vi "Parse Profile Status Response.vi"(8 "error in (no error)":errorcluster, 11 "Profile Status":string[](array[string])) -> (0 "error out":errorcluster, 3 "Profile Status":T1={"Profile State"=enum."Not Running", "Current Profile"=0, "Total Time Remaining"=0, "Total Steps"=0})   [LabVIEW 2018, in "F4T.lvlib" / "F4T.lvclass"]
uses:
  F4T.lvclass
  PPLs/Temp Chamber/Parent/Temp Chamber.lvlibp/Custom Controls/Profile Status.ctl
  PPLs/Temp Chamber/Parent/Temp Chamber.lvlibp/Custom Controls/Profile State.ctl
  PPLs/Temp Chamber/Parent/Temp Chamber.lvlibp/Temp Chamber.lvclass
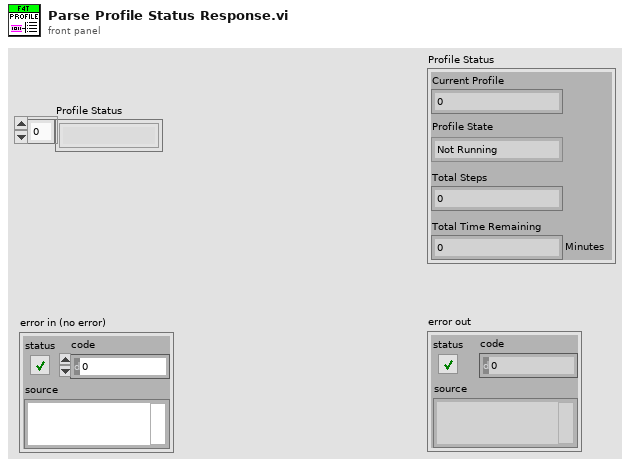
[diagram p1: front panel]
types:
  T1 = typedef "Temp Chamber.lvlibp/Temp Chamber.lvclass/Profile Status.ctl" = cluster{"Profile State":T2, "Current Profile":u32, "Total Time Remaining":u32, "Total Steps":u32}
  T2 = typedef "Temp Chamber.lvlibp/Temp Chamber.lvclass/Profile State.ctl" = enum16{"Running", "Not Running", "Paused", "Completed", "Terminated"}
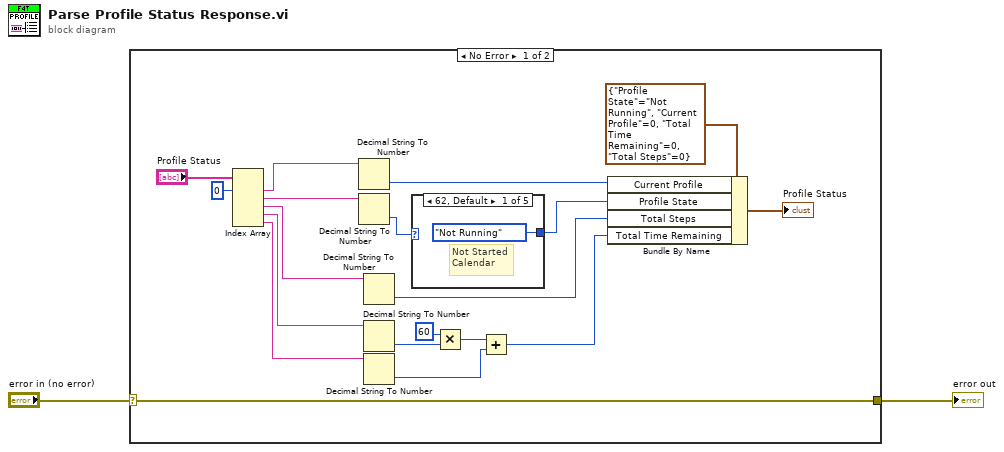
[diagram p0: block diagram]
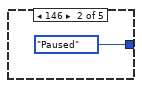
[diagram p2: hidden frame]
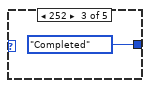
[diagram p3: hidden frame]
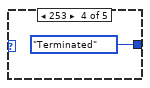
[diagram p4: hidden frame]
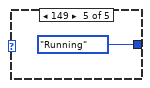
[diagram p5: hidden frame]
diagram:
  n1 = case shown="No Error" "error in (no error)" {
    selector: "error in (no error)" -> [w3 w27]
    tunnel: [w3 w27] -> w1
    frame No Error {
      n2 = Index Array(array="Profile Status", index #1=0 ("index")) -> (element #1=w20:string, element #2=w18:string, element #3=w15:string, element #4=w13:string, element #5=w12:string)  [unwired: 4 in]
      n3 = Decimal String To Number(string=w20) -> (number=w19:i32)  [unwired: 2 in, 1 out]
      n4 = Decimal String To Number(string=w18) -> (number=w17:i32)  [unwired: 2 in, 1 out]
      n5 = Decimal String To Number(string=w15) -> (number=w14:i32)  [unwired: 2 in, 1 out]
      n6 = Decimal String To Number(string=w13) -> (number=w11:i32)  [unwired: 2 in, 1 out]
      n7 = Decimal String To Number(string=w12) -> (number=w8:i32)  [unwired: 2 in, 1 out]
      n8 = case shown="62, Default" w17 {
        tunnel: [Profile_State."Not Running" ("Profile State") Profile_State."Paused" ("Profile State") Profile_State."Completed" ("Profile State") Profile_State."Terminated" ("Profile State") Profile_State."Running" ("Profile State")] -> w16
        frame 62, Default {
          # "Not Started\nCalendar"
        }
        frame 146 {
        }
        frame 252 {
        }
        frame 253 {
        }
        frame 149 {
        }
      }
      n9 = Multiply(x=60, y=w11) -> (x*y=w9:i32)
      n10 = Add(x=w9, y=w8) -> (x+y=w7:i32)
      n11 = Bundle By Name(cluster=T1 {"Profile State"=enum."Not Running", "Current Profile"=0, "Total Time Remaining"=0, "Total Steps"=0} ("Profile Status"), "Current Profile"=w19, "Profile State"=w16, "Total Steps"=w14, "Total Time Remaining"=w7) -> (→"Profile Status":T1)
    }
    frame Error {
    }
  }
  "error out" <- w1
